vi "ExternalCameraWindow.vi"(11 "Refnum in":T1) -> (3 "Refnum out":T1(plugin-control))   [LabVIEW 2011]
uses:
  <vilib>/vision/Image Controls.llb/IMAQ Image.ctl
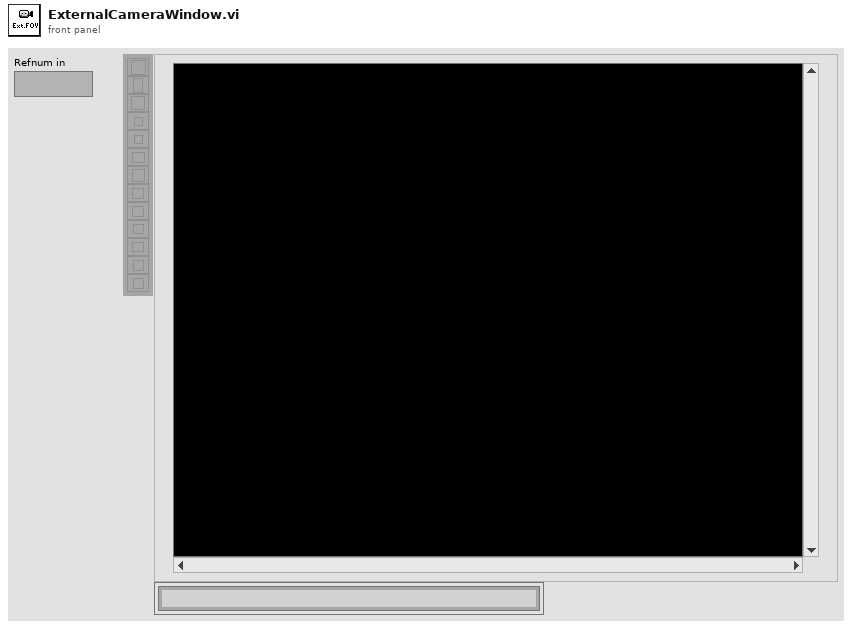
[diagram p1: front panel]
types:
  T1 = typedef "IMAQ Image.ctl" = refnum<image>
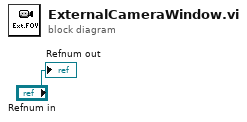
[diagram p0: block diagram]
diagram:
  "Refnum out" <- "Refnum in"
